vi "Switch.vi"(7 "array":bool[][](array[boolean]), 8 "Количество датчиков":i32, 9 "Номер иттерации":i32, 10 "task/channels in 2":refnum<k21>, 11 "task/channels in":refnum<k21>) -> (0 "Индекс переключаемого канала":i32, 1 "Что на самом деле":bool[](array[boolean]), 2 "task out 2":refnum<k21>, 3 "task out":refnum<k21>, 4 "Что следует из алгоритма":bool[](array[boolean]))   [LabVIEW 2018]
uses:
  <vilib>/DAQmx/read.llb/DAQmx Read (Digital 1D Bool NChan 1Samp 1Line).vi
  <vilib>/DAQmx/write.llb/DAQmx Write (Digital 1D Bool NChan 1Samp 1Line).vi
  <vilib>/DAQmx/miscellaneous.llb/DAQmx Fill In Error Info.vi
panel:
  # "Период перключения"
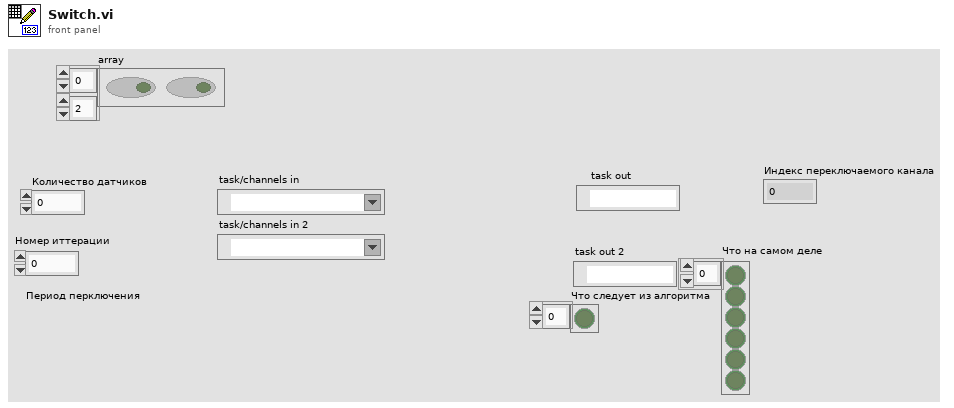
[diagram p1: front panel]
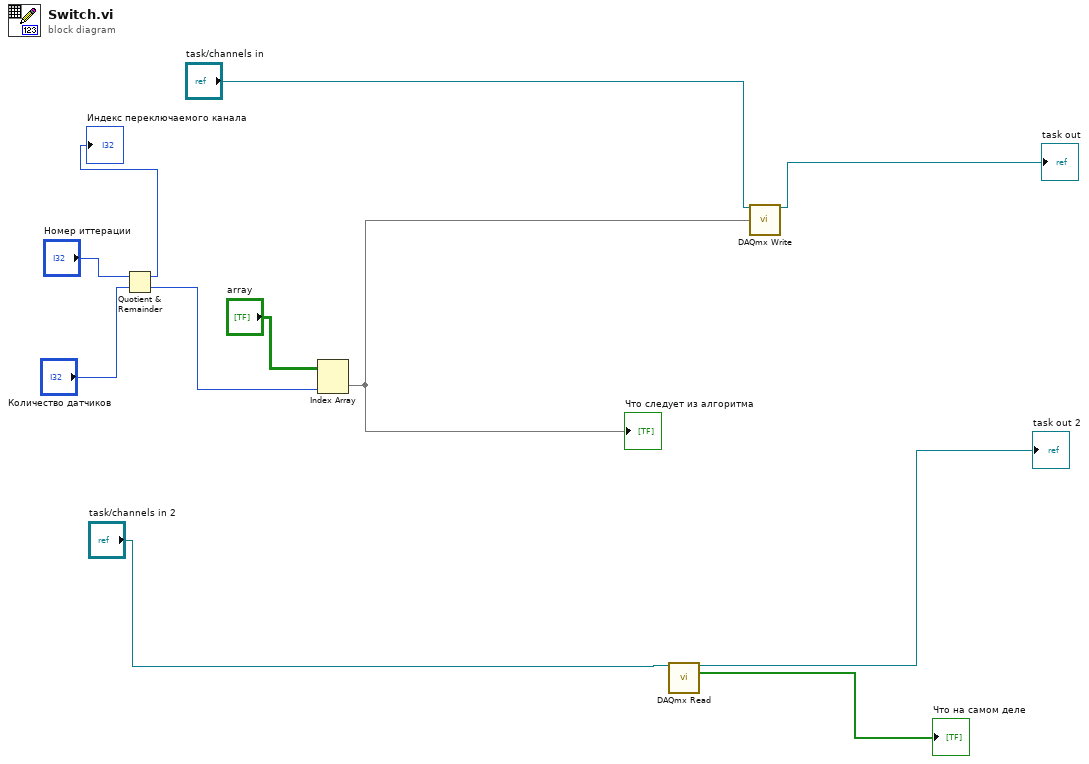
[diagram p0: block diagram]
diagram:
  n1 = Quotient & Remainder(x="Номер иттерации", y="Количество датчиков") -> (x-y*floor(x/y)=→"Индекс переключаемого канала":i32, floor(x/y)=w2:i32)
  n2 = Index Array(array="array", index (col)=w2) -> (element=w1:bool[])  [unwired: 1 in]
  "Что следует из алгоритма" <- w1
  n3 = call-poly <vilib>:"DAQmx Read.vi"("task/channels in"="task/channels in 2") -> ("task out"=→"task out 2":refnum<k21>, "data"=→"Что на самом деле":bool[])  [unwired: 12 in, 1 out]
  n4 = call-poly <vilib>:"DAQmx Write.vi"("task/channels in"="task/channels in", "data"=w1) -> ("task out"=→"task out":refnum<k21>)  [unwired: 11 in, 2 out]
